vi "New Assert Msg UT Main.vi"(8 "error in (no error)":errorcluster, 10 "Assert Message":T1, 11 "Standard Display Configuration in":refnum<class "Standard Display Configuration.lvclass">) -> (0 "error out":errorcluster, 1 "Assert Count":i32, 2 "Message Data Array":T1[](array[typedef]))   [LabVIEW 2016, in "Assert API Components.lvlib" / "Assert Display.lvlib" / "Main Display.lvlib" / "Standard Display Configuration.lvclass"]
uses:
  Standard Display Configuration.lvclass
  C:/Users/ukhornp/Documents/Projects/actor_assert_api/Core/Main Display/Display Configurations/Base Display Configuration.lvclass
  Assert API Components/Message Data.ctl
  Assert API Components/Failure Actions.ctl
  Assert API Components/VI References.ctl
  Base Display Configuration.lvclass/Base Display Configuration.ctl
  Standard Display Configuration.lvclass/Standard Display Configuration.ctl
  Base Display Configuration.lvclass
  Assert API Components/Assert API Components.lvlib
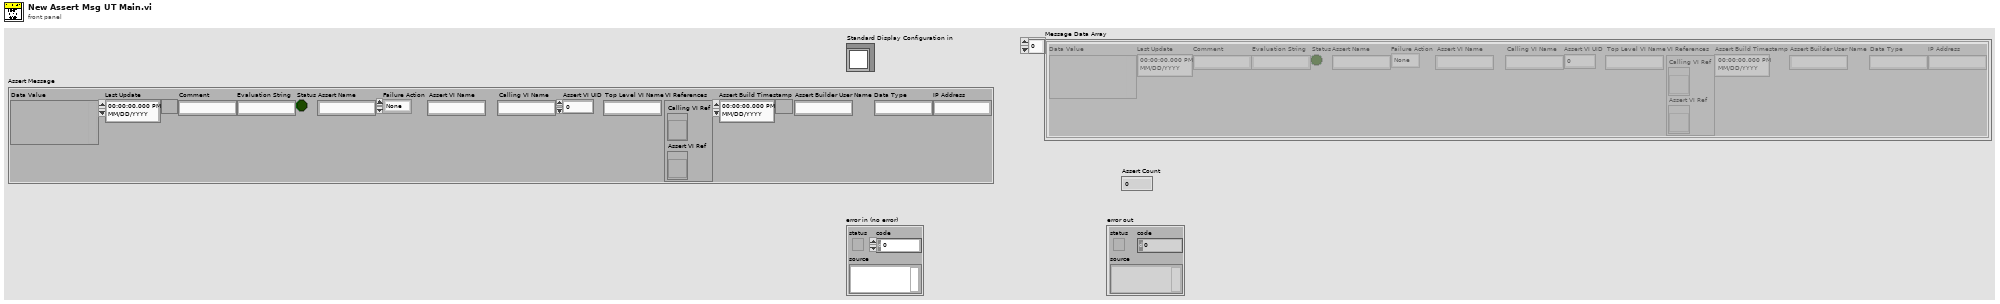
[diagram p1: front panel]
types:
  T1 = typedef "Assert API Components.lvlib/Message Data.ctl" = cluster{"Data Value":variant, "Last Update":timestamp, "Comment":string, "Evaluation String":string, "Status":bool, "Assert Name":string, "Failure Action":T2, "Assert VI Name":string, "Calling VI Name":string, "Assert VI UID":i32, "Top Level VI Name":string, "VI References":T3, "Assert Build Timestamp":timestamp, "Assert Builder User Name":string, "Data Type":string, "IP Address":string}
  T2 = typedef "Assert API Components.lvlib/Failure Actions.ctl" = enum16{"None", "Log To File", "Pause Execution", "Abort Execution"}
  T3 = typedef "Assert API Components.lvlib/VI References.ctl" = cluster{"Calling VI Ref":refnum<vi>, "Assert VI Ref":refnum<vi>}
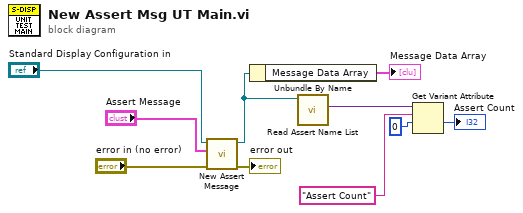
[diagram p0: block diagram]
diagram:
  n1 = call-dynamic "New Assert Message.vi"("error in (no error)"="error in (no error)", "Assert Message"="Assert Message", "Standard Display Configuration in"="Standard Display Configuration in") -> ("error out"=→"error out":errorcluster, "Standard Display Configuration out"=w5:refnum<class "Standard Display Configuration.lvclass">)  [unwired: 7 in]
  n2 = Unbundle By Name(w5) -> ("Message Data Array"=→"Message Data Array":T1[])
  n3 = call "Read Assert Name List.vi"("Base Display Configuration in"=w5) -> ("Assert Name List"=w4:variant)  [unwired: 10 in]
  n4 = Get Variant Attribute(Variant=w4, name="Assert Count", default value (empty Variant)=0) -> (value=→"Assert Count":i32)  [unwired: 1 in, 3 out]
